vi "CalibratedMultipleMeasurements.vi"(8 "error in":errorcluster, 9 "Time between calibrations (ms)":u32=1000, 10 "Time / ms (30000)":u32=30000, 11 "VISA resource name":refnum<visa-resource-name>) -> (0 "error out":errorcluster, 1 "Times / LSB":dbl[](array[numeric]), 2 "Times / s":dbl[](array[numeric]), 3 "VISA resource name out":refnum<visa-resource-name>)   [LabVIEW 2013, in "GP22_TDC_Arduinoed.lvlib"]
doc: "Take measurements for the given amount of time, returning an array of doubles and handling calibration automatically."
uses:
  GP22_TDC_Arduinoed.lvlib
  Globals.vi
  <vilib>/Analysis/NI_AALPro.lvlib
panel:
  out "Histogram Graph":T1(graph)
  out "Calibration / LSB":dbl[](array[numeric])
  out "MMProgress":u8(slide) scale=0.0..100.0
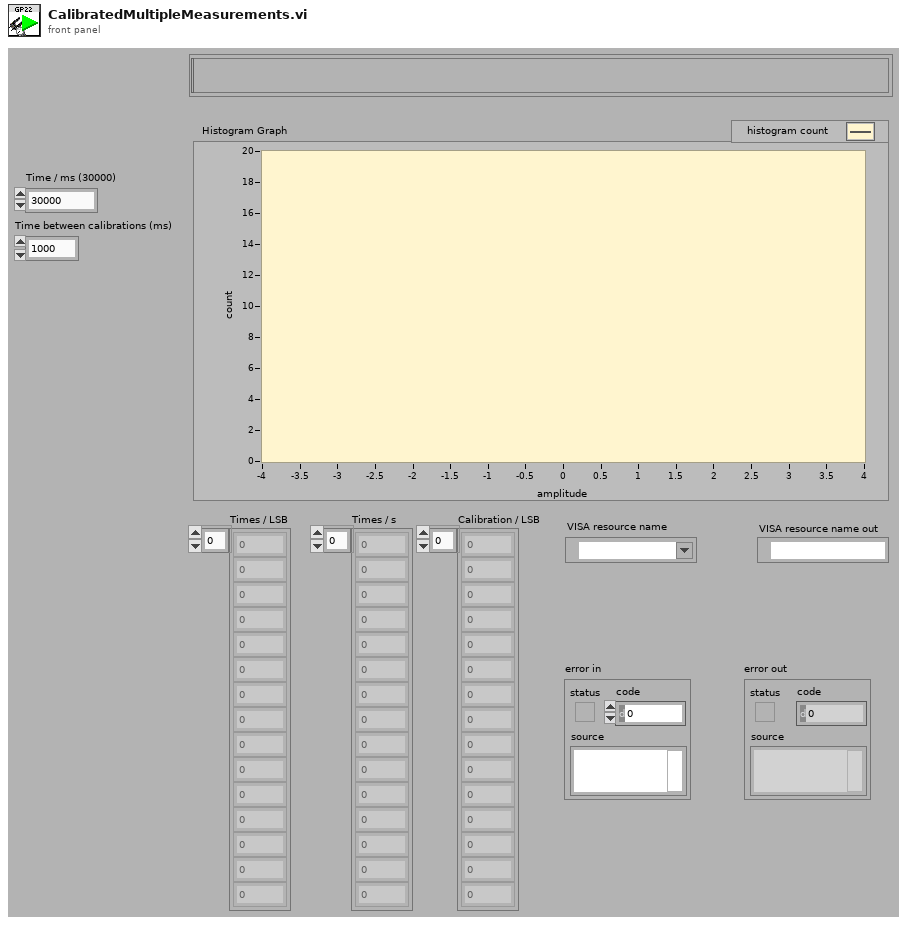
[diagram p1: front panel]
types:
  T1 = cluster{"X Values":dbl[], "Histogram: h(x)":i32[]}
  T2 = enum32{"Invalid", "Standard", "Closed", "Hidden", "Minimized", "Maximized"}
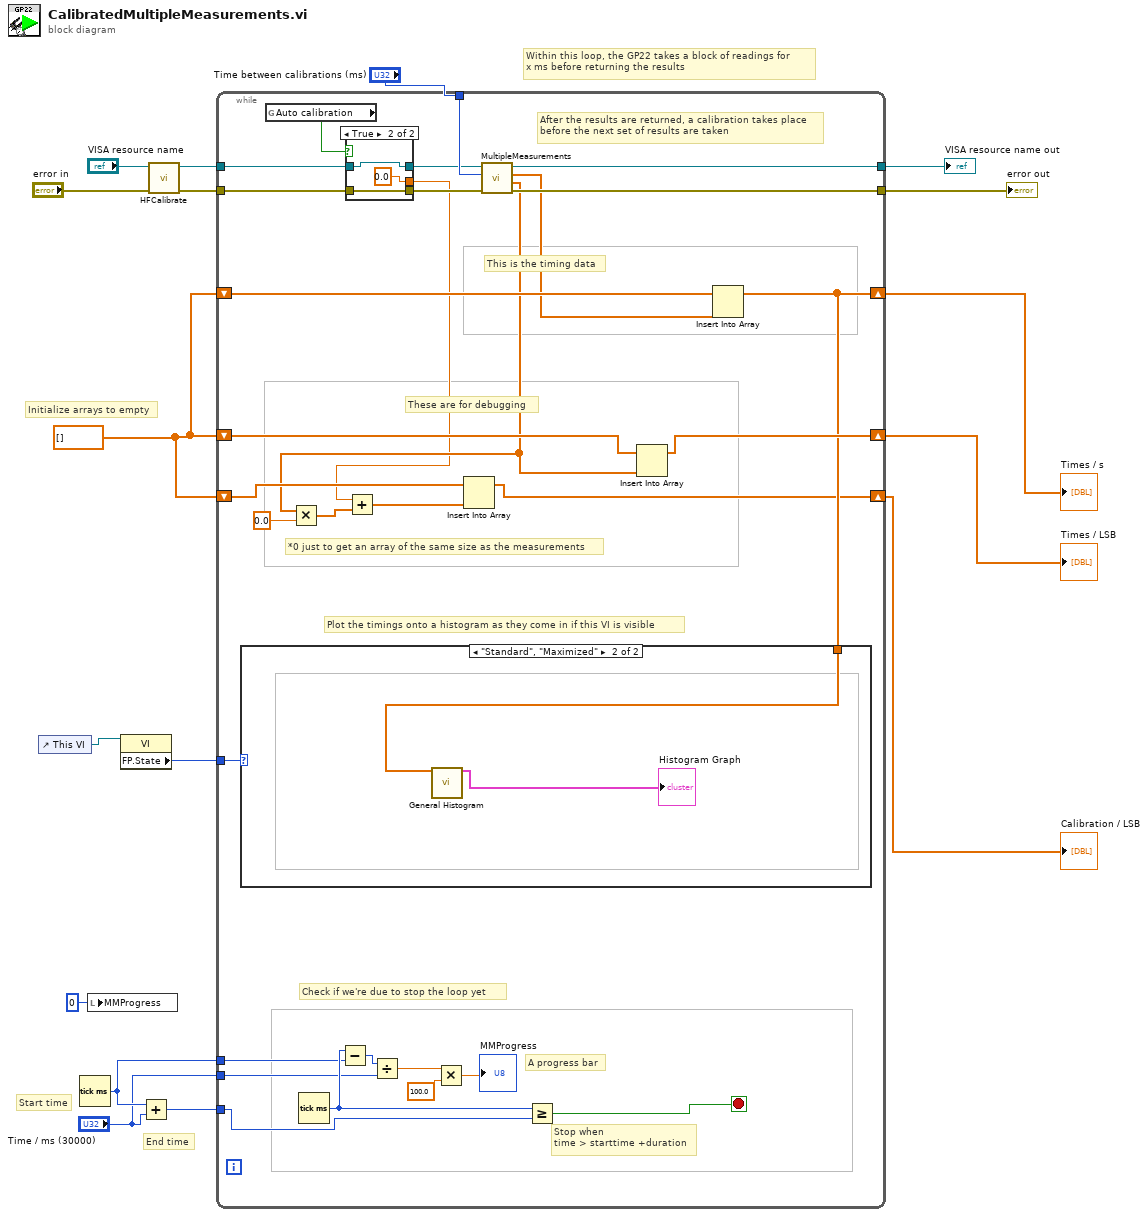
[diagram p0: block diagram]
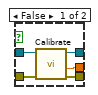
[diagram p3: hidden frame]
diagram:
  w8 = dbl[] []
  # "Initialize arrays to empty"
  # "Within this loop, the GP22 takes a block of readings for\nx ms before returning the results"
  # "End time"
  # "Start time"
  n1 = control-ref of="This VI"() -> (w7:refnum<vi>)
  n2 = Tick Count (ms)() -> (millisecond timer value=w15:u32)
  n3 = local write "MMProgress"(u8 0 ("MMProgress")) -> ()
  n4 = property class="VI"(reference=w7) -> ("FP.State"=w6:T2)  [unwired: 1 in, 2 out]
  n5 = Add(x=w15, y="Time / ms (30000)") -> (x+y=w17:u32)
  n6 = call "HFCalibrate.vi"("error in (no error)"="error in", "VISA resource name"="VISA resource name") -> ("error out"=w5:errorcluster, "VISA resource name out"=w4:refnum<visa-resource-name>)  [unwired: 5 in, 2 out]
  n7 = while {
    tunnel: [w47] -> w13
    tunnel: "Time between calibrations (ms)" -> [w46]
    tunnel: w5 -> [w43]
    tunnel: [w45] -> w12
    tunnel: w17 -> [w29]
    shift-right: [w28] -> w11
    shift-left: w8 -> [w40]
    shift-right: [w36] -> w10
    shift-left: w8 -> [w37]
    shift-right: [w20] -> w9
    shift-left: w8 -> [w35]
    tunnel: w15 -> [w26]
    tunnel: "Time / ms (30000)" -> [w24]
    tunnel: w6 -> [w19]
    tunnel: w4 -> [w18]
    stop <- w44 stop-if-true
    # "Plot the timings onto a histogram as they come in if this VI is visible"
    # "Check if we're due to stop the loop yet"
    # "A progress bar"
    # "These are for debugging"
    # "This is the timing data"
    # "After the results are returned, a calibration takes place\nbefore the next set of results are taken"
    # "*0 just to get an array of the same size as the measurements"
    # "Stop when \ntime > starttime +duration"
    n8 = global read "Globals.vi" "Auto calibration"() -> (w38:bool)
    n9 = Tick Count (ms)() -> (millisecond timer value=w27:u32)
    n10 = Subtract(x=w27, y=w26) -> (x-y=w25:u32)
    n11 = case shown="True" w38 {
      tunnel: w43 -> [w54 w57]
      tunnel: [w53 w57] -> w42
      tunnel: [w52 w55] -> w41
      tunnel: [w51 0.0 ("y")] -> w31
      tunnel: w18 -> [w50 w55]
      frame False {
        n12 = call "Calibrate.vi"("error in (no error)"=w54, "VISA resource name"=w50) -> ("error out"=w53:errorcluster, "output raw"=w51:dbl, "VISA resource name out"=w52:refnum<visa-resource-name>)  [unwired: 5 in, 1 out]
      }
      frame True {
      }
    }
    n13 = Divide(x=w25, y=w24) -> (x/y=w23:dbl)
    n14 = Multiply(x=w23, y=100.0) -> (x*y=→"MMProgress":dbl)
    n15 = call "MultipleMeasurements.vi"("error in (no error)"=w42, "Time in ms (30000)"=w46, "VISA resource name"=w41) -> ("error out"=w45:errorcluster, "Raw output"=w34:dbl[], "output/s"=w39:dbl[], "VISA resource name out"=w47:refnum<visa-resource-name>)  [unwired: 5 in]
    n16 = Multiply(x=w34, y=0.0) -> (x*y=w32:dbl[])
    n17 = Add(x=w31, y=w32) -> (x+y=w30:dbl[])
    n18 = Insert Into Array(array=w35, new element=w30) -> (w20:dbl[])  [unwired: 1 in]
    n19 = Greater Or Equal?(x=w27, y=w29) -> (x >= y?=w44:bool)
    n20 = Insert Into Array(array=w37, new element=w34) -> (w36:dbl[])  [unwired: 1 in]
    n21 = Insert Into Array(array=w40, new element=w39) -> (w28:dbl[])  [unwired: 1 in]
    n22 = case shown="\"Standard\", \"Maximized\"" w19 {
      tunnel: w28 -> [_ w49]
      frame "Invalid", Default {
        # "Do nothing here if this VI isn't visible"
      }
      frame "Standard", "Maximized" {
        n23 = call <vilib>:"General Histogram.vi"("X"=w49) -> ("Histogram Graph"=→"Histogram Graph":T1)  [unwired: 10 in, 4 out]
      }
    }
  }
  "VISA resource name out" <- w13
  "error out" <- w12
  "Times / s" <- w11
  "Times / LSB" <- w10
  "Calibration / LSB" <- w9
